vi "TEST - Filter Error Codes.vi"(8 "error in (no error)":errorcluster) -> (0 "error out":errorcluster, 2 "pass":bool)   [LabVIEW 2020]
uses:
  source/library/openg_error.lvlib
  source/library/Filter Error Codes/Filter Error Codes (Array).vi
  source/library/Filter Error Codes/Filter Error Codes (Scalar).vi
  source/library/Filter Error Codes/Filtered Error Details - Cluster.ctl
  <vilib>/addons/_JKI Toolkits/Caraya/classes/Assert/Assert.lvclass
  <vilib>/addons/_JKI Toolkits/Caraya/classes/Test/Test.lvclass
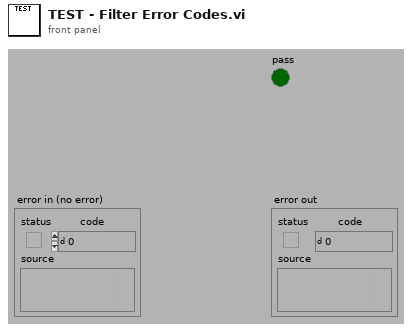
[diagram p1: front panel]
types:
  T1 = typedef "openg_error.lvlib/Filtered Error Details - Cluster.ctl" = cluster{"code":i32, "source":string}
  T2 = typedef "Filtered Error Details - Cluster.ctl" = cluster{"code":i32, "source":string}
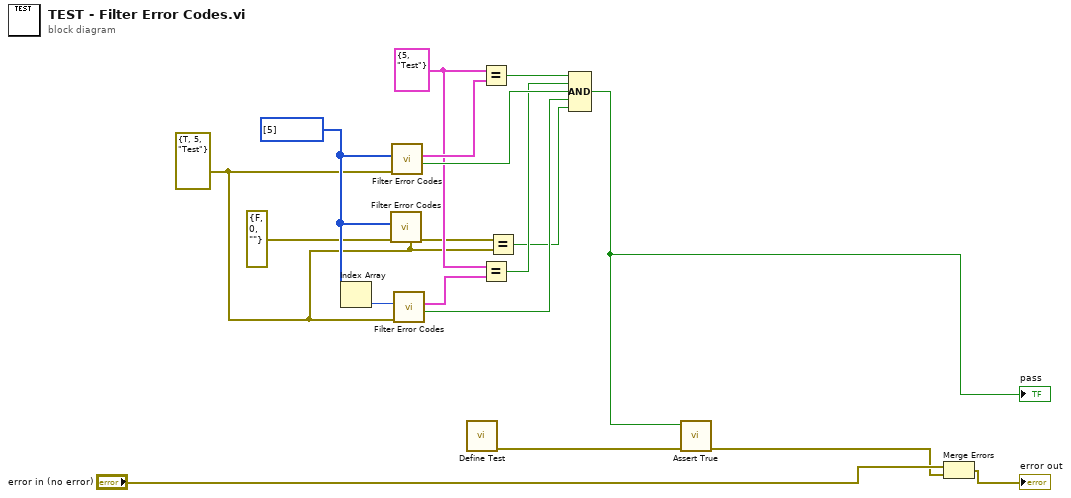
[diagram p0: block diagram]
diagram:
  w10 = T1 {"code"=5, "source"="Test"} ("Filtered Error Details")
  w7 = i32[] [5] ("Error Codes to Filter")
  w4 = errorcluster {"status"=TRUE, "code"=5, "source"="Test"} ("Error In")
  n1 = Index Array(array=w7) -> (element=w15:i32)  [unwired: 1 in]
  n2 = call-poly "Filter Error Codes.vi"("Upstream Error (optional)"=w4, "Error In"=errorcluster {"status"=FALSE, "code"=0, "source"=""}, "Error Codes to Filter"=w7) -> ("Error Out"=w5:errorcluster)  [unwired: 6 in, 2 out]
  n3 = call-poly "Filter Error Codes.vi"("Error In"=w4, "Error Codes to Filter"=w7) -> ("Error Filtered?"=w13:bool, "Filtered Error Details"=w12:T2)  [unwired: 7 in, 1 out]
  n4 = call-poly "Filter Error Codes.vi"("Error In"=w4, "Error Code to Filter"=w15) -> ("Error Filtered?"=w14:bool, "Filtered Error Details"=w11:T2)  [unwired: 7 in, 1 out]
  n5 = call <vilib>:"Define Test.vi"() -> ("error out"=w2:errorcluster)  [unwired: 11 in]
  n6 = Equal?(x=w10, y=w12) -> (x = y?=w9:bool)
  n7 = Equal?(x=w10, y=w11) -> (x = y?=w8:bool)
  n8 = Equal?(x=w5, y=w4) -> (x = y?=w3:bool)
  n9 = Compound Arithmetic op=AND(w9, w8, w13, w14, w3) -> (w18:bool)
  "pass" <- w18
  n10 = call <vilib>:"Assert True.vi"("error in (no error)"=w2, "True?"=w18) -> ("error out"=w1:errorcluster)  [unwired: 9 in]
  n11 = Merge Errors("error in (no error)", w1) -> (→"error out":errorcluster)
